vi "Digital Control.vi"() -> ()   [LabVIEW 2013]
uses:
  <vilib>/rvi/Emulation/niFpgaSctlEmulationGetInTimedLoop.vi
  <vilib>/rvi/Emulation/niFpgaEmulationReportErrorSimple.vi
  <vilib>/rvi/Emulation/niFpgaGetClockAttributes.vi
  <vilib>/rvi/eio/common/nirviEmuTemplateMethod_errors.vi
  <vilib>/rvi/Emulation/niFpgaCriticalErrorInLSC.vi
  <vilib>/rvi/Emulation/niFpgaProcessEmulError.vi
  <vilib>/eio/EIONode/EIONode.xnode
panel:
  in  "AO0":fxp<+/-,20,5>
  in  "RMC/DIO61":bool
  in  "Duty 2 (Ticks)":i32
  in  "Duty 1 (Ticks)":i32
  in  "Controller Period (ticks)":u32=40000
  in  "Frequency":sgl=18.0 min=18 max=22 step=1
  in  "PWM Period":u32=4000
  in  "Cycle Duty":i32
  in  "Enum":T1(ring)
  in  "Duty L":i32
  in  "Duty H":i32
  in  "Duty Ticks":i32
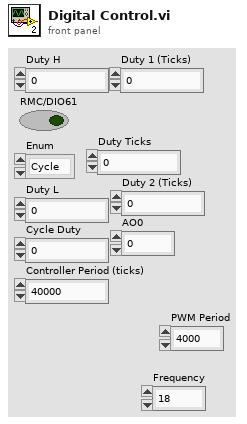
[diagram p1: front panel]
types:
  T1 = enum16{"Cycle", "Low Duty", "High Duty", "On", "Off"}
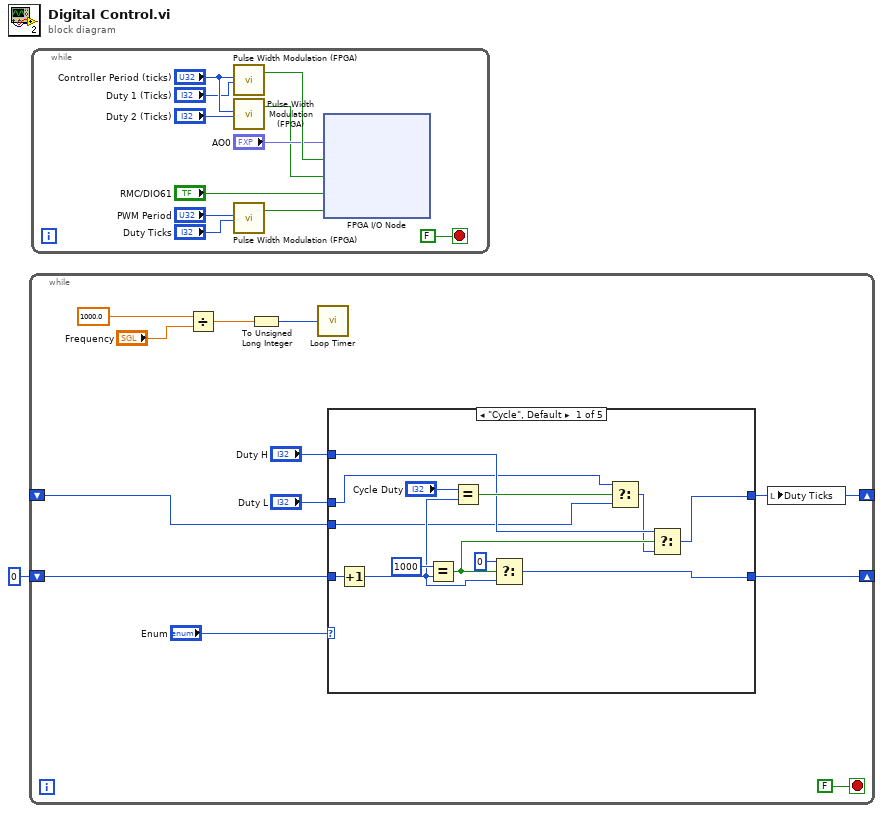
[diagram p0: block diagram]
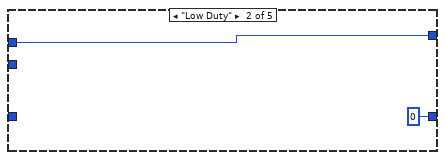
[diagram p2: hidden frame]
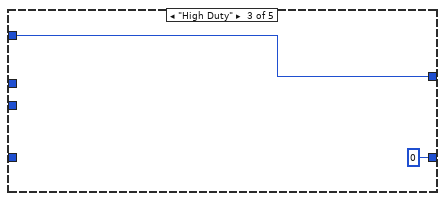
[diagram p3: hidden frame]
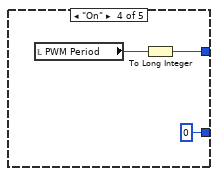
[diagram p4: hidden frame]
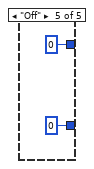
[diagram p5: hidden frame]
diagram:
  n1 = while {
    shift-right: [w8] -> _
    shift-left: 0 -> [w9]
    shift-right: [w7] -> _
    shift-left: _ -> [w6]
    stop <- FALSE stop-if-true
    n2 = Divide(x=sgl 1000.0, y="Frequency") -> (x/y=w2:sgl)
    n3 = To Unsigned Long Integer(number=w2) -> (unsigned 32bit integer=w5:u32)
    n4 = call "Loop Timer"("Count(uSec)"=w5) -> ()  [unwired: 1 out]
    n5 = case shown="\"Cycle\", Default" "Enum" {
      tunnel: "Duty H" -> [w18 _ w30 _ _]
      tunnel: "Duty L" -> [w17 w28 _ _ _]
      tunnel: [w14 w28 w30 w31 0 ("Duty H")] -> w7
      tunnel: w9 -> [w26 _ _ _ _]
      tunnel: [w23 0 0 0 0] -> w8
      tunnel: w6 -> [w16 _ _ _ _]
      frame "Cycle", Default {
        n6 = Increment(x=w26) -> (x+1=w21:i32)
        n7 = Equal?(x=1000 ("y"), y=w21) -> (x = y?=w20:bool)
        n8 = Equal?(x="Cycle Duty", y=w21) -> (x = y?=w19:bool)
        n9 = Select(t=0, s=w20, f=w21) -> (s? t:f=w23:i32)
        n10 = Select(t=w17, s=w19, f=w16) -> (s? t:f=w15:i32)
        n11 = Select(t=w18, s=w20, f=w15) -> (s? t:f=w14:i32)
      }
      frame "Low Duty" {
      }
      frame "High Duty" {
      }
      frame "On" {
        n12 = local read "PWM Period"() -> (w32:u32)
        n13 = To Long Integer(number=w32) -> (32bit integer=w31:i32)
      }
      frame "Off" {
      }
    }
    n14 = local write "Duty Ticks"(w7) -> ()
  }
  n15 = while {
    stop <- FALSE stop-if-true
    n16 = call "Pulse Width Modulation (FPGA).vi"("PWM Period (Ticks)"="Controller Period (ticks)", "PWM Duty Cycle (Ticks)"="Duty 1 (Ticks)") -> ("PWM DO"=w42:bool)  [unwired: 14 in, 3 out]
    n17 = call "Pulse Width Modulation (FPGA).vi"("PWM Period (Ticks)"="Controller Period (ticks)", "PWM Duty Cycle (Ticks)"="Duty 2 (Ticks)") -> ("PWM DO"=w36:bool)  [unwired: 14 in, 3 out]
    n18 = call "Pulse Width Modulation (FPGA).vi"("PWM Period (Ticks)"="PWM Period", "PWM Duty Cycle (Ticks)"="Duty Ticks") -> ("PWM DO"=w45:bool)  [unwired: 14 in, 3 out]
    n19 = xnode "FPGA I/O Node"("AO0"="AO0", "RMC/DIO0"=w42, "RMC/DIO1"=w36, "RMC/DIO61"="RMC/DIO61", "RMC/DIO62"=w45) -> ()  [unwired: 5 in, 5 out]
  }
